vi "ActionVIOnRecompile_InlineAsync.vi"(8 "error in":errorcluster, 9 "Timeout (ms)":u32, 10 "Runtime Configurable Section Path":string, 11 "Device Item Ref in":T1 format="%.0x") -> (0 "error out":errorcluster)   [LabVIEW 2020]
uses:
  <vilib>/NI VeriStand/Custom Device API/Custom Device Item Ref.ctl
  <vilib>/NI VeriStand/Custom Device API/Custom Device Channel Type.ctl
  <vilib>/NI VeriStand/Custom Device API/Block Data Reference.ctl
  <vilib>/NI VeriStand/Custom Device API/Data Reference.ctl
  <vilib>/NI VeriStand/Custom Device API/Get Item Property (U16).vi
  <vilib>/NI VeriStand/Custom Device API/Get Item Property (Variant).vi
  <vilib>/NI VeriStand/Execution/CustomDevice/NI VeriStand - Send Custom Device Message (Byte Array).vi
  <vilib>/NI VeriStand/Custom Device API/Custom Device API.lvlib
  <vilib>/NI/NIVS Inline Async API/_Data Access System Explorer/Data Access System Explorer.lvlib
  <vilib>/NI VeriStand/Execution/CustomDevice/NI_VS Custom Device ExecutionAPI.lvlib
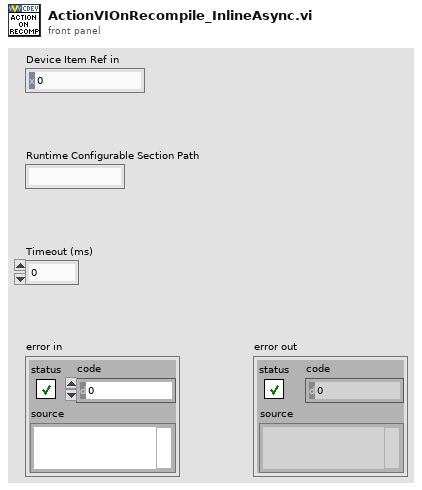
[diagram p1: front panel]
types:
  T1 = typedef "Custom Device API.lvlib/Custom Device Item Ref.ctl" = u64
  T2 = typedef "Custom Device API.lvlib/Custom Device Channel Type.ctl" = enum16{"Input", "Output"}
  T3 = cluster{"Name":string, "Type":enum16{"Output/Write", "Input/Read", "Input/ReadWrite"}, "VS Refs":T1[]}
  T4 = enum16{"Output/Write", "Input/Read", "Input/ReadWrite"}
  T5 = typedef "Custom Device API.lvlib/Block Data Reference.ctl" = cluster{"Data Reference":T6, "Offset":u64, "Length":u64}
  T6 = typedef "Custom Device API.lvlib/Data Reference.ctl" = i32
  T7 = cluster{"Read":cluster{"Refs":T5[], "Values":dbl[]}[], "Write":cluster{"Refs":T5[], "Values":dbl[]}[], "ReadWrite":cluster{"Refs":T6[], "Values":dbl[], "Reset Values":dbl[]}[], "LUT":variant}
  T8 = typedef "Custom Device API.lvlib/Custom Device Item Info.ctl" = cluster{"Name":string, "Is Channel":bool, "GUID":string, "Is Waveform":bool}
  T9 = cluster{"Name":string, "Type":enum16{"Output/Write", "Input/Read", "Input/ReadWrite"}, "VS Refs":T1[]}[]
  T10 = typedef "NI_VS Custom Device ExecutionAPI.lvlib/Custom Device Ref.ctl" = refnum<k24>
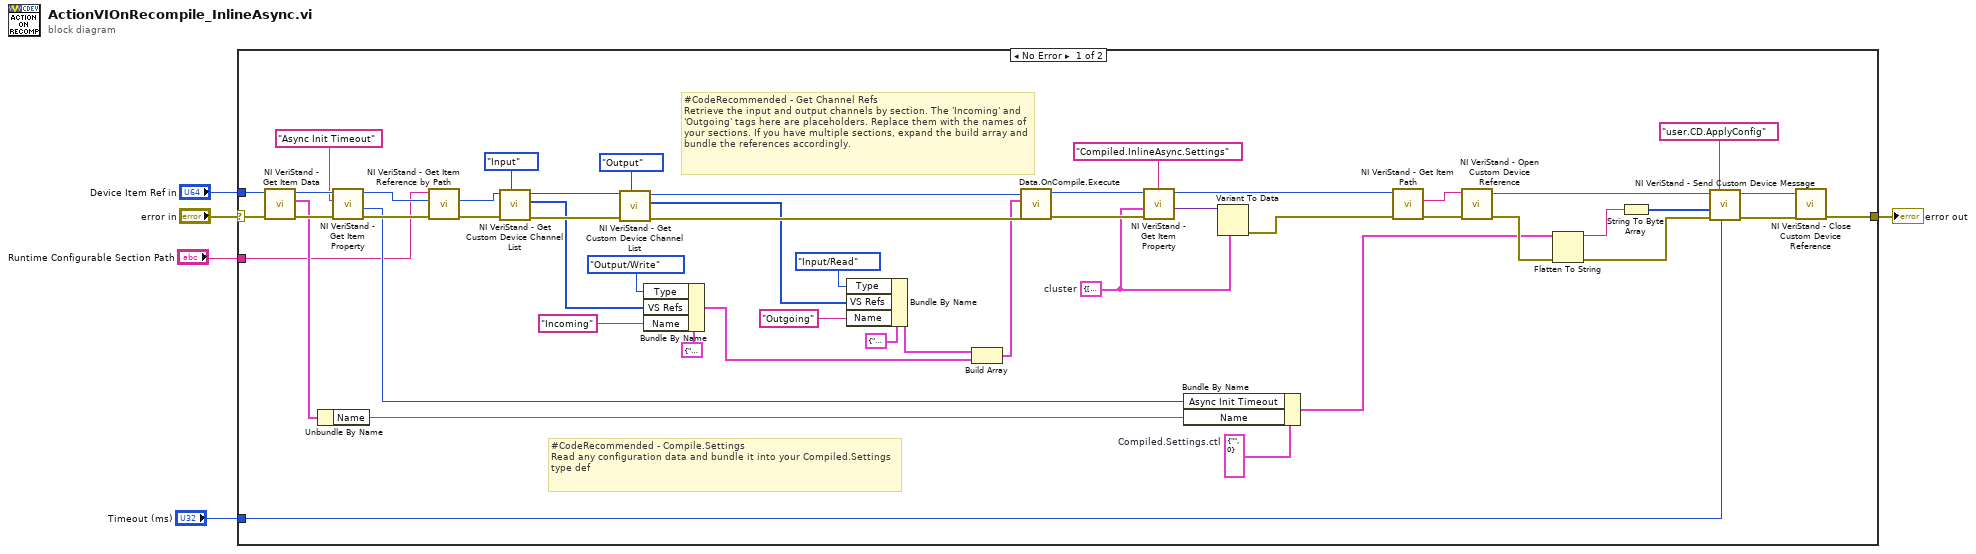
[diagram p0: block diagram]
diagram:
  n1 = case shown="No Error" "error in" {
    selector: "error in" -> [w56 w57]
    tunnel: [w45 w57] -> w4
    tunnel: "Device Item Ref in" -> [w43 _]
    tunnel: "Runtime Configurable Section Path" -> [w27 _]
    tunnel: "Timeout (ms)" -> [w7 _]
    frame No Error {
      w13 = T7 {"Read"=[], "Write"=[], "ReadWrite"=[], "LUT"=variant}  # cluster
      w19 = cluster{"Name":string, "Async Init Timeout":u16} {"Name"="", "Async Init Timeout"=0}  # Compiled.Settings.ctl
      # "#CodeRecommended - Get Channel Refs\nRetrieve the input and output channels by section. The 'Incoming' and 'Outgoing' tags here are placeholders. Replace them with the names of your sections. If you have multiple sections, expand the build array and bundle the references accordingly."
      # "#CodeRecommended - Compile.Settings\nRead any configuration data and bundle it into your Compiled.Settings type def"
      n2 = call <vilib>:"NI VeriStand - Get Item Data.vi"("error in (no error)"=w56, "Item Ref in"=w43) -> ("error out"=w55:errorcluster, "Item Info"=w42:T8, "Item Ref out"=w31:T1)  [unwired: 6 in, 1 out]
      n3 = Unbundle By Name(w42) -> ("Name"=w41:string)
      n4 = call-poly <vilib>:"NI VeriStand - Get Item Property.vi"("error in (no error)"=w55, "Property Name"="Async Init Timeout", "Item Ref in"=w31) -> ("error out"=w54:errorcluster, "Value"=w29:u16, "Item Ref out"=w28:T1)  [unwired: 5 in, 1 out]
      n5 = call <vilib>:"NI VeriStand - Get Item Reference by Path.vi"("error in (no error)"=w54, "Root Ref"=w28, "Item Path in"=w27) -> ("error out"=w53:errorcluster, "Item Ref"=w26:T1)  [unwired: 5 in, 2 out]
      n6 = call <vilib>:"NI VeriStand - Get Custom Device Channel List.vi"("Channel Type"=Custom_Device_Channel_Type."Input", "error in (no error)"=w53, "Device Ref in"=w26) -> ("error out"=w52:errorcluster, "Specified Channel Ref List"=w22:T1[], "Device Ref out"=w23:T1)  [unwired: 6 in]
      n7 = call <vilib>:"NI VeriStand - Get Custom Device Channel List.vi"("Channel Type"=Custom_Device_Channel_Type."Output", "error in (no error)"=w52, "Device Ref in"=w23) -> ("error out"=w51:errorcluster, "Specified Channel Ref List"=w21:T1[], "Device Ref out"=w20:T1)  [unwired: 6 in]
      n8 = Bundle By Name(cluster=T3 {"Name"="", "Type"=enum."Output/Write", "VS Refs"=[]} ("Group"), "Type"=T4."Output/Write", "VS Refs"=w22, "Name"="Incoming" ("Item Name")) -> (w32:T3)
      n9 = Bundle By Name(cluster=T3 {"Name"="", "Type"=enum."Output/Write", "VS Refs"=[]} ("Group"), "Type"=T4."Input/Read", "VS Refs"=w21, "Name"="Outgoing" ("Item Name")) -> (w37:T3)
      n10 = Build Array(w37, w32) -> (w35:T9)
      n11 = call <vilib>:"Data.OnCompile.Execute.vi"("error in"=w51, "VS Ref Groups"=w35, "Custom Device Ref"=w20) -> ("error out"=w48:errorcluster, "Custom Device Ref"=w15:T1)  [unwired: 7 in]
      n12 = call-poly <vilib>:"NI VeriStand - Get Item Property.vi"("error in (no error)"=w48, "Default Value"=w13, "Property Name"="Compiled.InlineAsync.Settings", "Item Ref in"=w15) -> ("Value"=w12:variant, "Item Ref out"=w6:T1)  [unwired: 4 in, 2 out]
      n13 = Bundle By Name(cluster=w19, "Async Init Timeout"=w29, "Name"=w41) -> (w11:cluster{"Name":string, "Async Init Timeout":u16})
      n14 = Variant To Data(type=w13, Variant=w12) -> (error out=w50:errorcluster)  [unwired: 1 in, 1 out]
      n15 = call <vilib>:"NI VeriStand - Get Item Path.vi"("error in (no error)"=w50, "Item Ref in"=w6) -> ("error out"=w49:errorcluster, "Path"=w18:string)  [unwired: 6 in, 2 out]
      n16 = call <vilib>:"NI VeriStand - Open Custom Device Reference.vi"("error in (no error)"=w49, "Custom Device Path"=w18) -> ("error out"=w47:errorcluster, "Custom Device"=w17:T10)  [unwired: 8 in]
      n17 = Flatten To String(anything=w11, error in (no error)=w47) -> (data string=w10:string, error out=w46:errorcluster)  [unwired: 2 in, 1 out]
      n18 = String To Byte Array(string=w10) -> (unsigned byte array=w9:u8[])
      n19 = call-poly <vilib>:"NI VeriStand - Send Custom Device Message.vi"("Timeout ms (5000)"=w7, "error in (no error)"=w46, "Data"=w9, "Command"="user.CD.ApplyConfig", "Custom Device in"=w17) -> ("error out"=w44:errorcluster, "Custom Device out"=w8:T10)  [unwired: 4 in, 1 out]
      n20 = call <vilib>:"NI VeriStand - Close Custom Device Reference.vi"("error in (no error)"=w44, "Custom Device"=w8) -> ("error out"=w45:errorcluster)  [unwired: 9 in]
    }
    frame Error {
    }
  }
  "error out" <- w4
